vi "shuntRead.vi"(8 "error in (no error)":errorcluster, 10 "stop":bool, 11 "Data Cluster":T1) -> ()   [LabVIEW 2026, in "Acquisition.lvlib"]
uses:
  Acquisition.lvlib
  <vilib>/DAQmx/read.llb/DAQmx Read (Analog 1D DBL 1Chan NSamp).vi
  Hardware Configuration.ctl
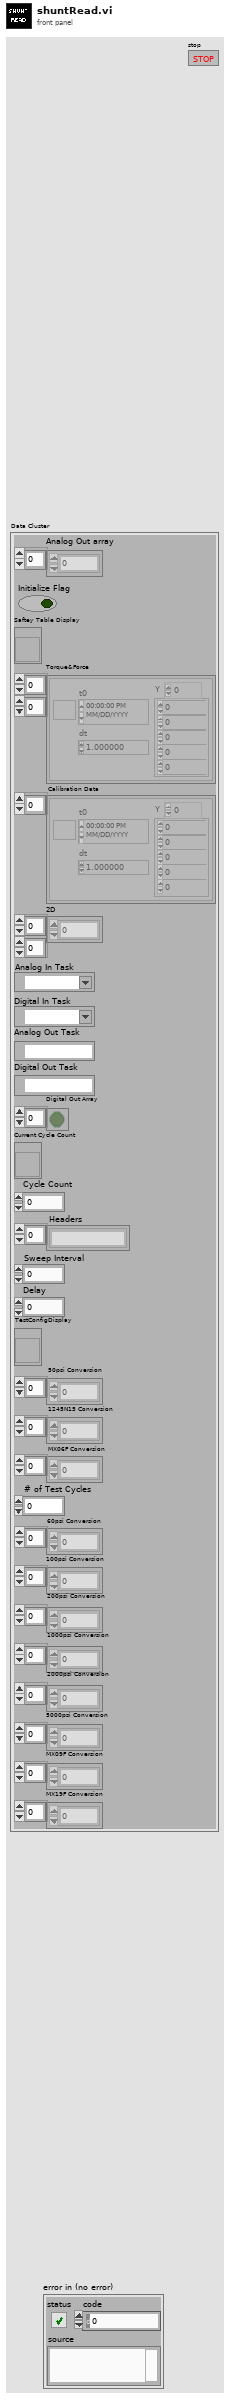
[diagram p1: front panel]
types:
  T1 = typedef "Acquisition.lvlib/Hardware Configuration.ctl" = cluster{"Analog Out array":dbl[], "Initialize Flag":bool, "Saftey Table Display":refnum<vi>, "Torque&Force":waveform(dbl)[][], "Calibration Data":waveform(dbl)[], "2D":dbl[][], "Analog In Task":refnum<k21>, "Digital In Task":refnum<k21>, "Analog Out Task":refnum<k21>, "Digital Out Task":refnum<k21>, "Digital Out Array":bool[], "Current Cycle Count":refnum<vi>, "Cycle Count":u64, "Headers":string[], "Sweep Interval":u64, "Delay":u64, "TestConfigDisplay":refnum<vi>, "50psi Conversion":dbl[], "1245N15 Conversion":dbl[], "MX06F Conversion":dbl[], "# of Test Cycles":u64, "60psi Conversion":dbl[], "100psi Conversion":dbl[], "200psi Conversion":dbl[], "1000psi Conversion":dbl[], "2000psi Conversion":dbl[], "5000psi Conversion":dbl[], "MX09F Conversion":dbl[], "MX19F Conversion":dbl[]}
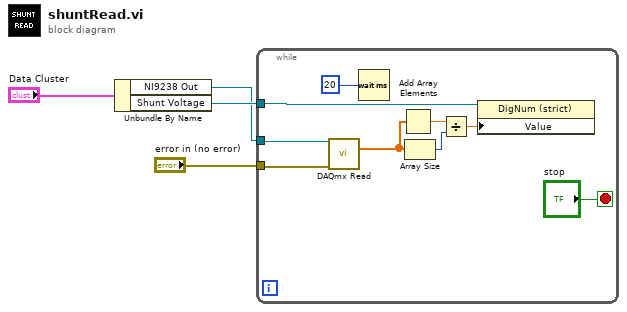
[diagram p0: block diagram]
diagram:
  n1 = Unbundle By Name("Data Cluster") -> ("NI9238 Out"=w2:refnum<k21>, "Shunt Voltage"=w4:refnum<vi>)
  n2 = while {
    tunnel: w2 -> [w8]
    tunnel: "error in (no error)" -> [w7]
    tunnel: w4 -> [w6]
    stop <- "stop" stop-if-true
    n3 = call-poly <vilib>:"DAQmx Read.vi"("task/channels in"=w8, "error in"=w7) -> ("data"=w10:dbl[])  [unwired: 11 in, 2 out]
    n4 = Wait (ms)(milliseconds to wait=u32 20) -> ()  [unwired: 1 out]
    n5 = Add Array Elements(numeric array=w10) -> (sum=w12:dbl)
    n6 = Array Size(array=w10) -> (size(s)=w9:i32)
    n7 = Divide(x=w12, y=w9) -> (x/y=w11:dbl)
    n8 = property class="DigNum (strict)"(reference=w6, "Value"=w11) -> ()  [unwired: 1 in, 2 out]
  }
